vi "Get Tree Item by Left Cell String.vi"(10 "Left Cell String":string, 11 "Tree Items":T1(array[cluster])) -> (3 "Item":T2)   [LabVIEW 2020, in "Result Model Test Enumeration.lvclass"]
uses:
  Result Model Test Enumeration.lvclass
  Result Model Test Enumeration.lvclass/Result Model Test Enumeration.ctl
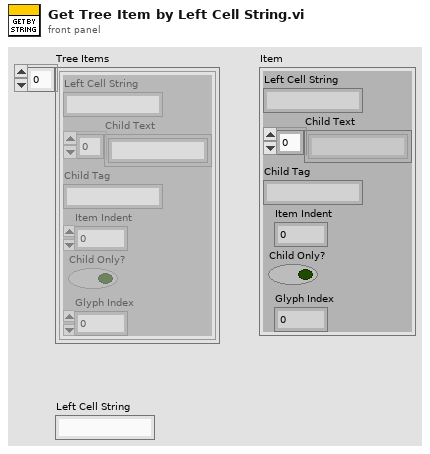
[diagram p1: front panel]
types:
  T1 = cluster{"Left Cell String":string, "Child Text":string[], "Child Tag":string, "Item Indent":i32, "Child Only?":bool, "Glyph Index":i32}[]
  T2 = cluster{"Left Cell String":string, "Child Text":string[], "Child Tag":string, "Item Indent":i32, "Child Only?":bool, "Glyph Index":i32}
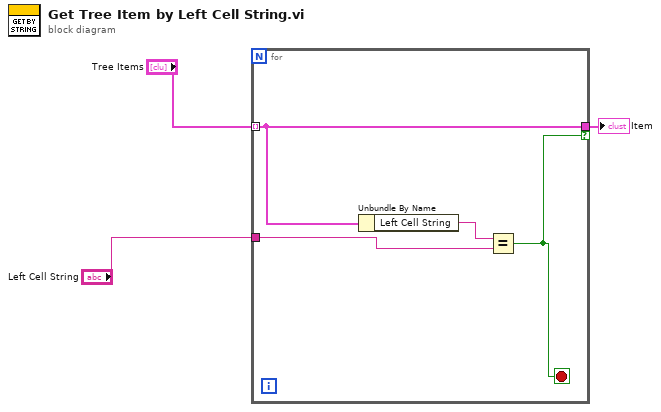
[diagram p0: block diagram]
diagram:
  n1 = for {
    tunnel: "Tree Items" -> [w5] mode=indexing
    tunnel: "Left Cell String" -> [w7]
    tunnel: [w5] -> w3 if=w4
    stop <- w4 stop-if-true
    n2 = Unbundle By Name(w5) -> ("Left Cell String"=w6:string)
    n3 = Equal?(x=w6, y=w7) -> (x = y?=w4:bool)
  }
  "Item" <- w3
